vi "add indices to control pairs.vi"(6 "fpga res type":T1, 8 "fpga resource":refnum<k20>, 9 "data index":i32, 10 "data type":T3, 11 "pairs in":T2[](array[typedef])) -> (3 "pairs out":T2[](array[typedef]))   [LabVIEW 2015, in "io runtime.lvclass"]
uses:
  io runtime.lvclass
  <vilib>/NI/Tag Bus/tag/Data Type.ctl
  control index set.ctl
  configuration/fpga resource supported data types.ctl
  <vilib>/NI/Tag Bus/tag/tag descriptor.lvclass
  configuration/io configuration.lvclass
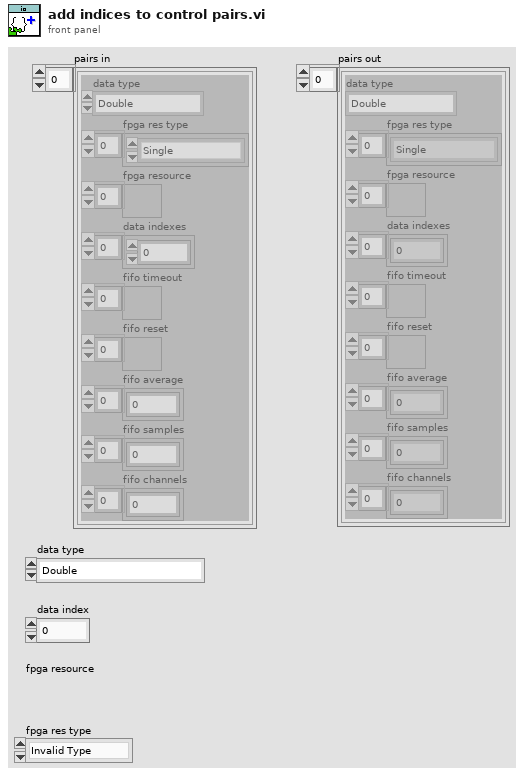
[diagram p1: front panel]
types:
  T1 = typedef "io configuration.lvclass/fpga resource supported data types.ctl" = enum16{"Invalid Type", "Single", "I64", "I32", "I16", "I8", "U64", "U32", "U16", "U8", "Boolean", "FXP I,20,5", "FXP I,24,5", "FXP I,24,10", "Fifo 1023,I16"}
  T2 = typedef "io runtime.lvclass/control index set.ctl" = cluster{"data type":T3, "fpga res type":T1[], "fpga resource":refnum<k20>[], "data indexes":i32[], "fifo timeout":refnum<k20>[], "fifo reset":refnum<k20>[], "fifo average":i32[], "fifo samples":u32[], "fifo channels":u32[]}
  T3 = typedef "tag bus.lvlib/tag descriptor.lvclass/Data Type.ctl" = enum16{"Double", "Single", "I64", "I32", "I16", "I8", "U64", "U32", "U16", "U8", "Boolean", "String", "Array of Double", "Array of Single", "Array of I64", "Array of I32", "Array of I16", "Array of I8", "Array of U64", "Array of U32", "Array of U16", "Array of U8", "Array of Boolean", "Array of String"}
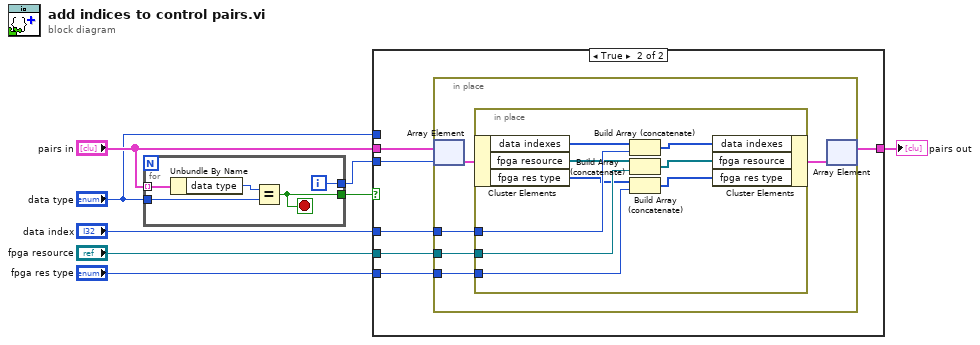
[diagram p0: block diagram]
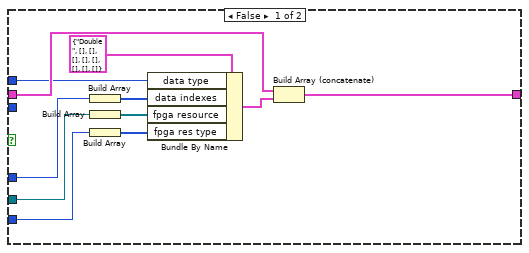
[diagram p2: hidden frame]
diagram:
  n1 = for {
    tunnel: "pairs in" -> [w13] mode=indexing
    tunnel: "data type" -> [w11]
    tunnel: [w10] -> w2
    tunnel: [w9] -> w8
    i -> [w10]
    stop <- w9 stop-if-true
    n2 = Unbundle By Name(w13) -> ("data type"=w12:T3)
    n3 = Equal?(x=w12, y=w11) -> (x = y?=w9:bool)
  }
  n4 = case shown="True" w8 {
    tunnel: "pairs in" -> [w24 w30]
    tunnel: [w23 w29] -> w6
    tunnel: w2 -> [_ w28]
    tunnel: "fpga resource" -> [w19 w27]
    tunnel: "data index" -> [w17 w26]
    tunnel: "data type" -> [w20 _]
    tunnel: "fpga res type" -> [w15 w25]
    frame False {
      n5 = Build Array(w17) -> (w18:i32[])
      n6 = Build Array(w19) -> (w16:refnum<k20>[])
      n7 = Build Array(w15) -> (w14:T1[])
      n8 = Bundle By Name(cluster=T2 {"data type"=enum."Double", "fpga res type"=[], "fpga resource"=[], "data indexes"=[], "fifo timeout"=[], "fifo reset"=[], "fifo average"=[], "fifo samples"=[], "fifo channels"=[]} ("control index set"), "data type"=w20, "data indexes"=w18, "fpga resource"=w16, "fpga res type"=w14) -> (w21:T2)
      n9 = Build Array (concatenate)(w24, w21) -> (w23:T2[])
    }
    frame True {
      n10 = in-place {
        in-place-border: w27 -> [w33]
        in-place-border: w26 -> [w32]
        in-place-border: w25 -> [w31]
        n11 = in-place-array #1(w30, w28) -> (w35:T2)
        n12 = in-place {
          in-place-border: w33 -> [w42]
          in-place-border: w32 -> [w41]
          in-place-border: w31 -> [w36]
          n13 = in-place-cluster #2(w35) -> ("data indexes"=w44:i32[], "fpga resource"=w40:refnum<k20>[], "fpga res type"=w38:T1[])
          n14 = Build Array (concatenate)(w44, w41) -> (w43:i32[])
          n15 = Build Array (concatenate)(w40, w42) -> (w39:refnum<k20>[])
          n16 = Build Array (concatenate)(w38, w36) -> (w37:T1[])
          n17 = in-place-cluster #2("data indexes"=w43, "fpga resource"=w39, "fpga res type"=w37) -> (w34:T2)
        }
        n18 = in-place-array #1(w34) -> (w29:T2[])  [unwired: 1 out]
      }
    }
  }
  "pairs out" <- w6
